vi "prog test connection.vi"() -> ()   [LabVIEW 2009]
uses:
  <vilib>/real-time/rtutility.llb/subVIs/RT Target Information.ctl
  <vilib>/real-time/rtutility.llb/subVIs/IP Settings.ctl
  <vilib>/real-time/rtutility.llb/RT Get Target Information (IP).vi
  <vilib>/real-time/NI_Real-Time Libraries.lvlib
panel:
  out "Connection Status":string
  in  "target address":string="10.0.35.206"
  out "target information":T1 {"serial number" format="%x"}
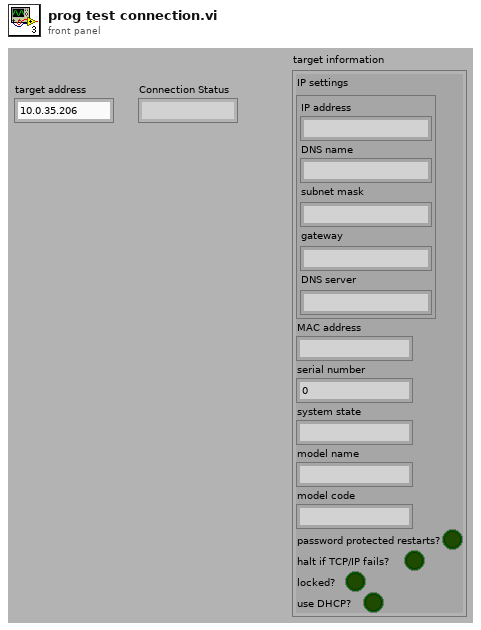
[diagram p1: front panel]
types:
  T1 = typedef "NI_Real-Time Libraries.lvlib/RT Target Information.ctl" = cluster{"IP settings":T2, "MAC address":string, "serial number":u32, "system state":string, "model name":string, "model code":string, "password protected restarts?":bool, "halt if TCP/IP fails?":bool, "locked?":bool, "use DHCP?":bool}
  T2 = typedef "NI_Real-Time Libraries.lvlib/IP Settings.ctl" = cluster{"IP address":string, "DNS name":string, "subnet mask":string, "gateway":string, "DNS server":string}
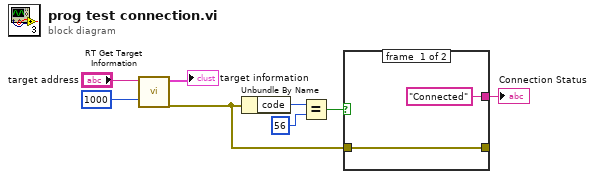
[diagram p0: block diagram]
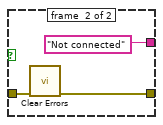
[diagram p2: hidden frame]
diagram:
  n1 = call-poly <vilib>:"RT Get Target Information.vi"("timeout in ms (4000)"=1000, "target address"="target address") -> ("error out"=w3:errorcluster, "target information"=→"target information":T1)  [unwired: 8 in]
  n2 = Unbundle By Name(w3) -> ("code"=w6:i32)
  n3 = Equal?(x=w6, y=56) -> (x = y?=w4:bool)
  n4 = case shown="True" w4 {
    tunnel: w3 -> [w9 w13]
    tunnel: ["Connected" "Not connected"] -> w2
    tunnel: [w9 w11] -> _
    frame #0 {
    }
    frame #1 {
      n5 = call <vilib>:"Clear Errors.vi"("error in (no error)"=w13) -> ("error out"=w11:errorcluster)  [unwired: 6 in]
    }
  }
  "Connection Status" <- w2
